vi "读取工作目录路径.vi"(8 "error in (no error)":errorcluster caption="错误输入（无错误）", 11 "EPUB输入":refnum<class "EPUB.lvclass">) -> (0 "error out":errorcluster caption="错误输出", 2 "工作目录路径":path, 3 "EPUB输出":refnum<class "EPUB.lvclass">)   [LabVIEW 2016, in "EPUB.lvclass"]
uses:
  EPUB.lvclass
  EPUB.lvclass/EPUB.ctl
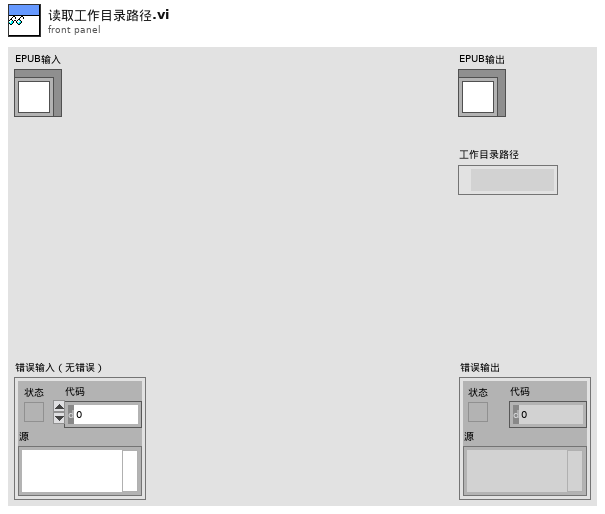
[diagram p1: front panel]
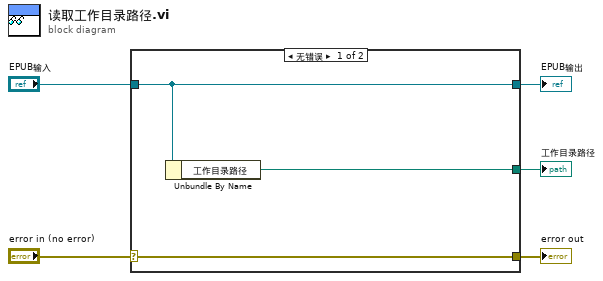
[diagram p0: block diagram]
diagram:
  n1 = case shown="无错误" "error in (no error)" {
    selector: "error in (no error)" -> [w8 w9]
    tunnel: [w8 w9] -> w4
    tunnel: [w7 w10] -> w2
    tunnel: "EPUB输入" -> [w7 w10]
    tunnel: [w6 _] -> w1
    frame No Error {
      n2 = Unbundle By Name(w7) -> ("工作目录路径"=w6:path)
    }
    frame Error {
    }
  }
  "error out" <- w4
  "EPUB输出" <- w2
  "工作目录路径" <- w1
